vi "dataset.free.vi"(8 "error in":errorcluster, 11 "Dataset":refnum<class "Dataset.lvclass">) -> (0 "error out":errorcluster)   [LabVIEW 2020, in "Dataset.lvclass"]
doc: "Releases the handle and its associated resources."
uses:
  Dataset.lvclass
  Dataset.lvclass/Dataset.ctl
  client.lvlib
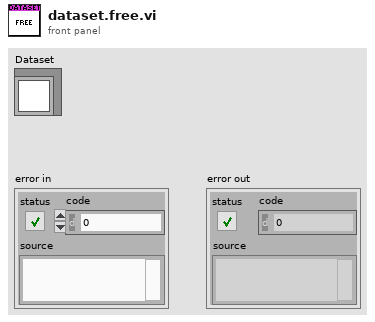
[diagram p1: front panel]
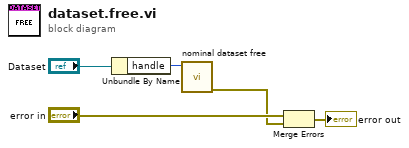
[diagram p0: block diagram]
diagram:
  n1 = Unbundle By Name("Dataset") -> ("handle"=w5:i32)
  n2 = call "nominal dataset free.vi"("dataset"=w5) -> ("error out"=w2:errorcluster)  [unwired: 9 in, 1 out]
  n3 = Merge Errors("error in", w2) -> (→"error out":errorcluster)
